vi "get_guide_points.vi"(8 "error in (no error)":errorcluster, 11 "TrajectoryDL110420DoubleCircle in":refnum<class "TrajectoryDL110420DoubleCircle.lvclass">) -> (0 "error out":errorcluster, 2 "guide points":refnum<class "SpaceVector.lvclass">[](array[class]), 3 "TrajectoryDL110420DoubleCircle out":refnum<class "TrajectoryDL110420DoubleCircle.lvclass">)   [LabVIEW 2010, in "TrajectoryDL110420DoubleCircle.lvclass"]
uses:
  TrajectoryDL110420DoubleCircle.lvclass
  common/classes/SpaceVector/SpaceVector/SpaceVector.lvclass
  TrajectoryDL110420DoubleCircle.lvclass/TrajectoryDL110420DoubleCircle.ctl
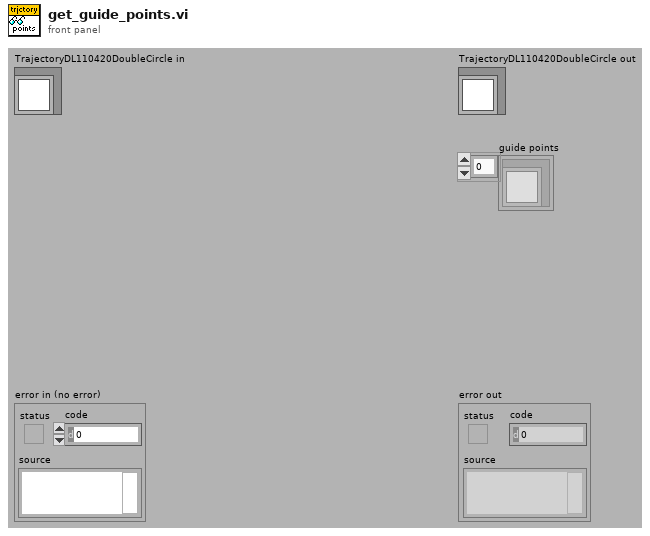
[diagram p1: front panel]
types:
  T1 = typedef "ROImicrons_cluster.ctl" = cluster{"Global Rectangle":dbl[unit][], "Contours":cluster{"Contour Type":u32, "ROI Type":u32, "Points":dbl[unit][]}[]}
  T2 = cluster{"Contour Type":u32, "ROI Type":u32, "Points":dbl[unit][]}[]
  T3 = cluster{"Points[0]":dbl[unit], "Points[1]":dbl[unit]}
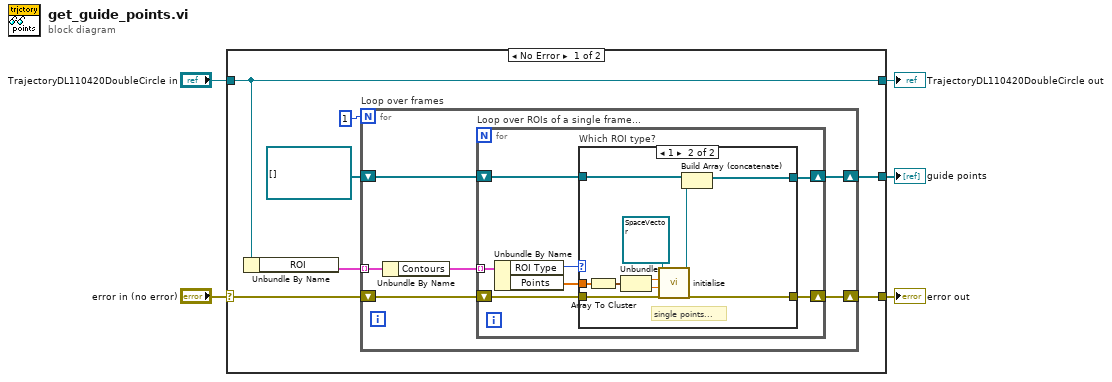
[diagram p0: block diagram]
diagram:
  n1 = case shown="No Error" "error in (no error)" {
    selector: "error in (no error)" -> [w12 w39]
    tunnel: [w11 w39] -> w4
    tunnel: [w6 w38] -> w2
    tunnel: "TrajectoryDL110420DoubleCircle in" -> [w6 w38]
    tunnel: [w7 _] -> w1
    frame No Error {
      n2 = Unbundle By Name(w6) -> ("ROI"=w8:T1[])
      n3 = for "Loop over frames" {
        N: 1 -> [_]
        tunnel: w8 -> [w18] mode=indexing
        shift-right: [w16] -> w11
        shift-left: w12 -> [w17]
        shift-right: [w13] -> w7
        shift-left: refnum<class "SpaceVector.lvclass">[] [] -> [w14]
        n4 = Unbundle By Name(w18) -> ("Contours"=w15:T2)
        n5 = for "Loop over ROIs of a single frame..." {
          shift-right: [w21] -> w16
          shift-left: w17 -> [w22]
          tunnel: w15 -> [w25] mode=indexing
          shift-right: [w20] -> w13
          shift-left: w14 -> [w19]
          n6 = Unbundle By Name(w25) -> ("ROI Type"=w24:u32, "Points"=w23:dbl[unit][])
          n7 = case "Which ROI type?" shown="1" w24 {
            tunnel: w23 -> [_ w37]
            tunnel: w22 -> [w27 w35]
            tunnel: [w27 w34] -> w21
            tunnel: [w26 w31] -> w20
            tunnel: w19 -> [w26 w30]
            frame Default {
              # "not supported..."
            }
            frame 1 {
              # "single points..."
              n8 = Array To Cluster(array=w37) -> (cluster=w36:T3)
              n9 = Unbundle(w36) -> ("Points[0]"=w33:dbl[unit], "Points[1]"=w32:dbl[unit])
              n10 = call "initialise.vi"("error in (no error)"=w35, "y"=w32, "x"=w33, "SpaceVector in"=refnum<class "SpaceVector.lvclass"> refnum ("SpaceVector.lvclass")) -> ("error out"=w34:errorcluster, "SpaceVector out"=w28:refnum<class "SpaceVector.lvclass">)  [unwired: 6 in]
              n11 = Build Array (concatenate)(w30, w28) -> (w31:refnum<class "SpaceVector.lvclass">[])
            }
          }
        }
      }
    }
    frame Error {
    }
  }
  "error out" <- w4
  "TrajectoryDL110420DoubleCircle out" <- w2
  "guide points" <- w1
